vi "Set DPM Range.vi"(8 "error in (no error)":errorcluster, 10 "Measurement Voltage":string, 11 "Measurement in":refnum<class "Measurement.lvclass">) -> (0 "error out":errorcluster, 3 "Measurement out":refnum<class "Measurement.lvclass">)   [LabVIEW 2015, in "Measurement.lvclass"]
uses:
  Measurement.lvclass
  CBTF Applications/Driver Board Testing/Main/Application/Application/Class/typedefs/Instrument Selector -- Enum.ctl
  Classes/Instruments/Digital Power Meter/Digital Power Meter/Class/Digital Power Meter.lvclass
  Test Class/Test Class.lvclass
  Classes/Application/Class/Application.lvclass
  Classes/Test Recipe/Class/Test Recipe.lvclass
  CBTF Applications/Driver Board Testing/Main/Application/Application/Class/Driver Board Test.lvclass
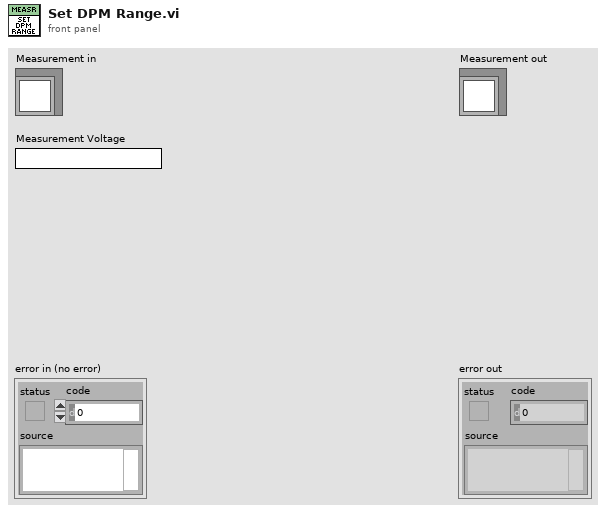
[diagram p1: front panel]
types:
  T1 = typedef "Driver Board Test.lvlib/Driver Board Test.lvclass/Instrument Selector -- Enum.ctl" = enum16{"ACPS1", "ACPS2", "DCPS1", "DCPS2", "DCPS3", "DCLoad1", "DCLoad2", "DPM1", "DPM2", "Switch1", "PXI1Slot2", "PXI1Slot3", "cDAQ1Mod5", "cDAQ1Mod6", "cDAQ1Mod7", "cDAQ1Mod8", "cDAQ1Mod1", "cDAQ1Mod2", "cDAQ1Mod3", "cDAQ1Mod4", "cDAQ2Mod1", "cDAQ2Mod2", "cDAQ2Mod3", "cDAQ2Mod4"}
  T2 = typedef "Application.lvlib/App Properties.lvclass/Class Properties -- Cluster.ctl" = cluster{"UUT Info":T3[], "Test Information":refnum<vi>, "Test Complete Event":refnum<user-event>, "Shop Floor System":refnum<class "Shop Floor System.lvclass">, "Gold Board":refnum<class "Golden Board.lvclass">, "Test Recipe":refnum<class "Test Recipe.lvclass">, "Instruments":refnum<class "Instrument.lvclass">[], "Mode":T4, "Test Results":T5[], "Station Config":refnum<class "Station Config.lvclass">}
  T3 = typedef "Application.lvlib/App Properties.lvclass/UUT Reference -- Cluster.ctl" = cluster{"Serial Number Reference":refnum<vi>, "Status Message Reference":refnum<vi>}
  T4 = typedef "Application.lvlib/Application.lvclass/Op Mode -- Enum.ctl" = u16
  T5 = typedef "Application.lvlib/App Properties.lvclass/Test Result -- Cluster.ctl" = cluster{"Position":i32, "Pass":bool, "Fail Codes":string}
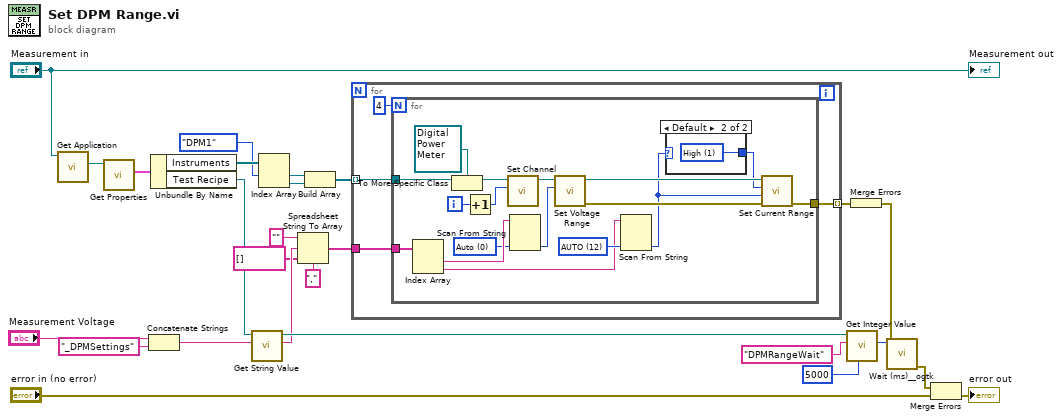
[diagram p0: block diagram]
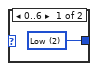
[diagram p2: hidden frame]
diagram:
  n1 = call "Get Application.vi"("Test Class in"="Measurement in") -> ("Application.lvlib:Application.lvclass"=w23:refnum<class "Application.lvclass">)  [unwired: 9 in, 1 out]
  n2 = call "Get Properties.vi"("Acrobat Template in"=w23) -> ("Class Properties"=w24:T2)  [unwired: 8 in, 2 out]
  n3 = Concatenate Strings("Measurement Voltage", "_DPMSettings" ("string")) -> (w18:string)
  n4 = Unbundle By Name(w24) -> ("Instruments"=w22:refnum<class "Instrument.lvclass">[], "Test Recipe"=w19:refnum<class "Test Recipe.lvclass">)
  n5 = call "Get String Value.vi"("Name"=w18, "Test Recipe in"=w19) -> ("Value"=w9:string, "Test Recipe out"=w11:refnum<class "Test Recipe.lvclass">)  [unwired: 6 in, 2 out]
  n6 = Index Array(array=w22, index #1=Instrument_Selector_--_Enum."DPM1" ("Instrument")) -> (element #1=w15:refnum<class "Instrument.lvclass">, element #2=w16:refnum<class "Instrument.lvclass">)  [unwired: 1 in]
  n7 = Spreadsheet String To Array(delimiter (Tab)=",", format string="", spreadsheet string=w9, array type (2D Dbl)=string[] [] ("format string")) -> (array=w6:string[])
  n8 = Build Array(w15, w16) -> (w10:refnum<class "Instrument.lvclass">[])
  n9 = for {
    tunnel: w10 -> [w30] mode=indexing
    tunnel: w6 -> [w29]
    tunnel: [w28] -> w4 mode=indexing
    n10 = for {
      N: 4 -> [_]
      tunnel: w30 -> [w47]
      tunnel: w29 -> [w44]
      tunnel: [w34] -> w28
      i -> [w36]
      w40 = u32 12 items=["AUTO"=12, "20A"=11, "5A"=10, "2A"=9, "0.5A"=8, "0.2A"=7, "0.05A"=6, "0.02A"=5, "0.005A"=4, "0.1V"=3, "0.05V"=2, "0.025V"=1, "0.01V"=0] ("Current Range In")
      w42 = 0 items=["Auto", "V600", "V300", "V150", "V60", "V30", "V15"] ("Voltage Range")
      n11 = Index Array(array=w44) -> (element #1=w43:string, element #2=w33:string)  [unwired: 2 in]
      n12 = To More Specific Class(target class=refnum<class "Digital Power Meter.lvclass"> refnum ("Digital Power Meter.lvlib:Digital Power Meter.lvclass"), reference=w47) -> (specific class reference=w38:refnum<class "Digital Power Meter.lvclass">)  [unwired: 1 in, 1 out]
      n13 = Increment(x=w36) -> (x+1=w35:i32)
      n14 = call-dynamic "Set Channel.vi"("Channel"=w35, "Acrobat Template in"=w38) -> ("Acrobat Template out"=w37:refnum<class "Digital Power Meter.lvclass">)  [unwired: 8 in, 1 out]
      n15 = Scan From String(input string=w43, default 1=w42) -> (output 1=w41:i32)  [unwired: 3 in, 3 out]
      n16 = call-dynamic "Set Voltage Range.vi"("Voltage Range"=w41, "Acrobat Template in"=w37) -> ("error out"=w39:errorcluster, "Acrobat Template out"=w45:refnum<class "Digital Power Meter.lvclass">)  [unwired: 8 in]
      n17 = Scan From String(input string=w33, default 1=w40) -> (output 1=w32:u32)  [unwired: 3 in, 3 out]
      n18 = case shown="Default" w32 {
        tunnel: [w48 w49] -> w31
        frame 0..6 {
          w48 = u32 2 items=["Auto", "High", "Low"] ("Shunt Range In")
        }
        frame Default {
          w49 = u32 1 items=["Auto", "High", "Low"] ("Shunt Range In")
        }
      }
      n19 = call-dynamic "Set Current Range.vi"("error in (no error)"=w39, "Current Range In"=w32, "Shunt Range In"=w31, "Acrobat Template in"=w45) -> ("error out"=w34:errorcluster)  [unwired: 6 in, 1 out]
    }
  }
  n20 = call "Get Integer Value.vi"("Default Value"=u32 5000 ("milliseconds to wait"), "Name"="DPMRangeWait", "Test Recipe in"=w11) -> ("Value"=w14:i32)  [unwired: 5 in, 3 out]
  n21 = Merge Errors(w4) -> (w2:errorcluster)
  n22 = call <userlib>:"Wait (ms)__ogtk.vi"("error in (no error)"=w2, "milliseconds to wait"=w14) -> ("error out"=w1:errorcluster)  [unwired: 8 in, 1 out]
  n23 = Merge Errors(w1, "error in (no error)") -> (→"error out":errorcluster)
  "Measurement out" <- "Measurement in"
